vi "Test SMO Facade.vi"() -> ()   [LabVIEW 2019]
doc: "JKI State Machine Objects (SMO) 1.3.0.56\nJKI - JKI\nCopyright (c) 2017, JKI"
uses:
  SMO/SMO.lvclass
  SMO/Typedefs/SMOState --Enum.ctl
  Facade/SMOFacade.lvclass
panel:
  in  "Test Mismatch Inputs":bool
  out "Default Input":variant
  out "Method Prototype":string
  in  "Component URL":u16(ring) items=["System", "System/Subsystem"]
  in  "Invoke Method":bool
  in  "Public Methods":u16(ring) items=["CheckAccessibility", "Get GUID", "Get Name", "Get Qualified Name", "GetGUID", "GetName", "GetQualifiedName", "GetReserveState", "GetState", "Set Process Kill timeout", "WaitForStateChange", "is StateMachineObject", "isStateMachineObject"]
  out "Final Error":errorcluster
  out "return":variant
  out "Invoke Method Error":errorcluster
  # "Returns\n>>>>"
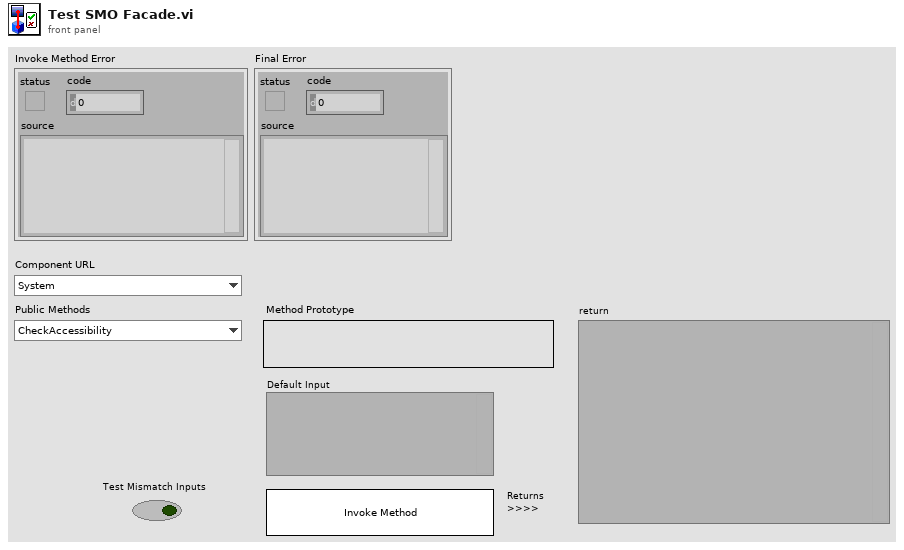
[diagram p1: front panel]
types:
  T1 = typedef "SMO.lvclass/Public Events.ctl" = cluster{"Error":refnum<user-event>, "State":refnum<user-event>, "Reserve State":refnum<user-event>}
  T2 = typedef "SMO.lvclass/SMOState --Enum.ctl" = enum16{"unknown", "Created", "Started", "Stopped"}
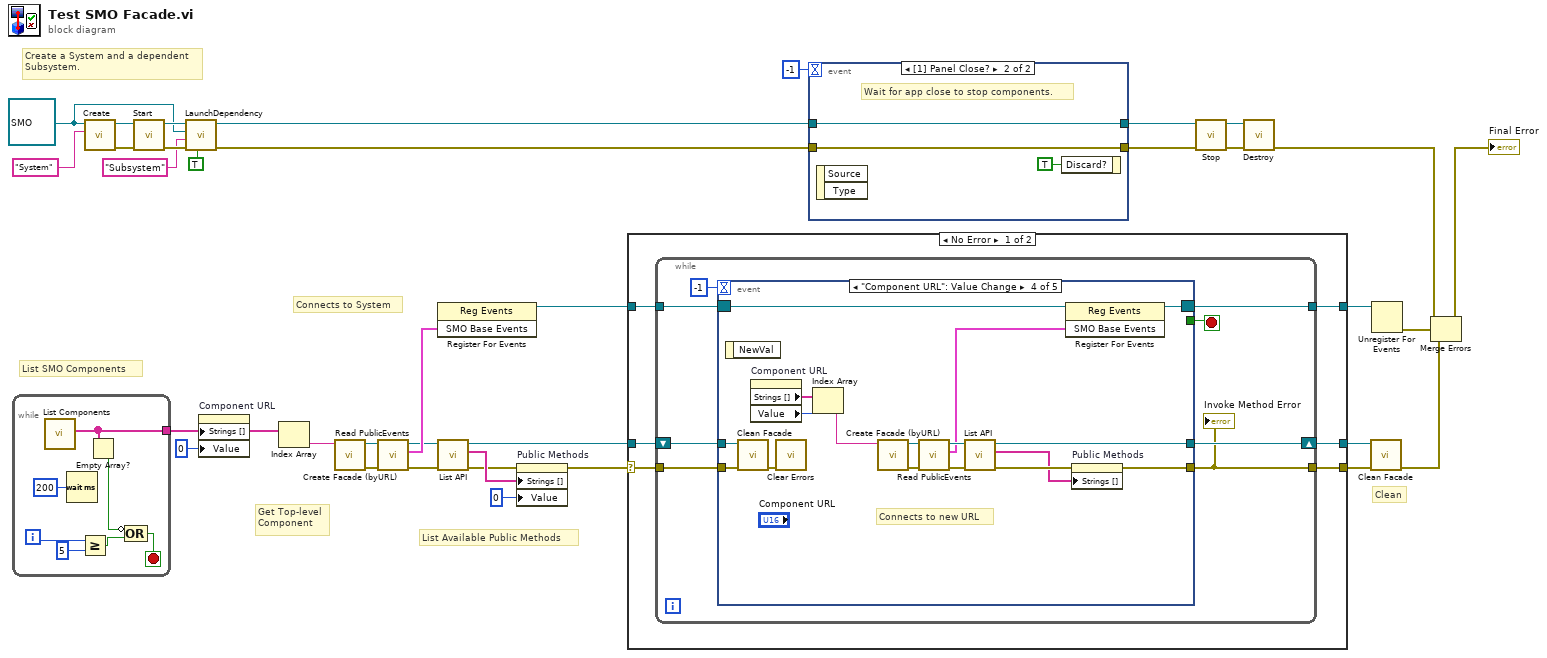
[diagram p0: block diagram]
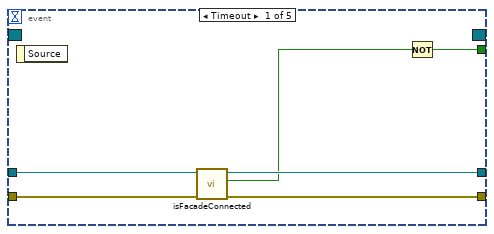
[diagram p2: hidden frame]
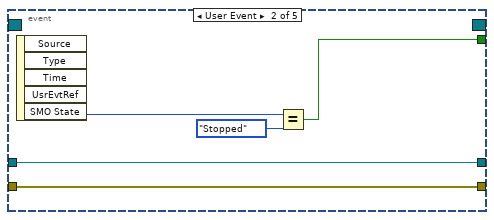
[diagram p3: hidden frame]
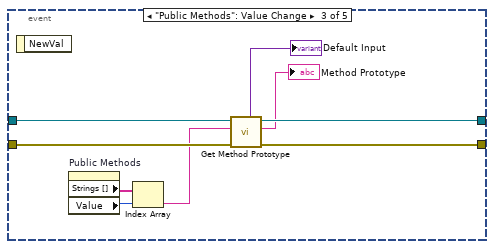
[diagram p4: hidden frame]
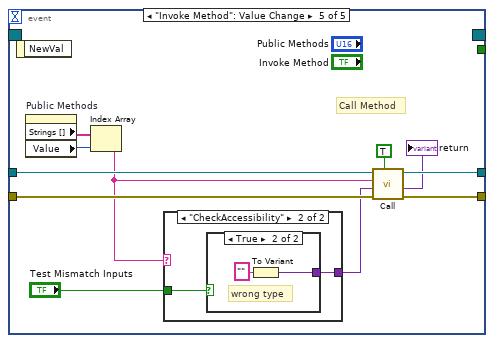
[diagram p5: hidden frame]
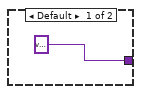
[diagram p6: hidden frame]
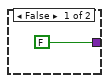
[diagram p7: hidden frame]
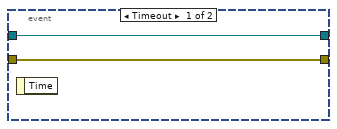
[diagram p9: hidden frame]
diagram:
  w15 = refnum<class "SMO.lvclass"> refnum ("SMO")
  # "List SMO Components"
  # "Get Top-level\nComponent"
  # "Connects to System"
  # "Clean"
  # "List Available Public Methods"
  # "Create a System and a dependent\nSubsystem."
  n1 = while {
    tunnel: [w37] -> w2
    i -> [w42]
    stop <- w39 stop-if-true
    n2 = call "List Components.vi"() -> ("Components"=w37:string[])  [unwired: 9 in, 2 out]
    n3 = Wait (ms)(milliseconds to wait=u32 200) -> ()  [unwired: 1 out]
    n4 = Greater Or Equal?(x=w42, y=5) -> (x >= y?=w40:bool)
    n5 = Empty Array?(array=w37) -> (empty?=w38:bool)
    n6 = Compound Arithmetic op=OR(invert w38, w40) -> (w39:bool)
  }
  n7 = call "Create.vi"("Subsystem Name (optional)"="System", "SMO"=w15) -> ("error out"=w23:errorcluster, "SMO out"=w24:refnum<class "SMO.lvclass">)  [unwired: 7 in, 1 out]
  n8 = call "Start.vi"("error in (no error)"=w23, "SMO"=w24) -> ("error out"=w21:errorcluster, "SMO out"=w22:refnum<class "SMO.lvclass">)  [unwired: 8 in]
  n9 = call "LaunchDependency.vi"("Shared Resource"=TRUE, "error in (no error)"=w21, "Dependency Name"="Subsystem" ("Subsystem Name (optional)"), "Dependency Type"=w15, "SMO in"=w22) -> ("error out"=w11:errorcluster, "SMO out"=w12:refnum<class "SMO.lvclass">)  [unwired: 3 in, 2 out]
  n10 = property on="Component URL" class="Ring (strict)"("Strings []"=w2, "Value"=u16 0) -> ()  [unwired: 2 in, 2 out]
  n11 = Index Array(array=w2) -> (element=w3:string)  [unwired: 1 in]
  n12 = call "Create Facade (byURL).vi"("URL"=w3) -> ("error out"=w4:errorcluster, "SMOFacade out"=w5:refnum<class "SMOFacade.lvclass">)  [unwired: 9 in]
  n13 = call "Read PublicEvents.vi"("error in (no error)"=w4, "SMOFacade in"=w5) -> ("error out"=w19:errorcluster, "SMO Base Events"=w18:T1, "SMOFacade out"=w17:refnum<class "SMOFacade.lvclass">)  [unwired: 7 in]
  n14 = register-events(w18) -> (reference out=w27:refnum<event-registration>)  [unwired: 2 in, 1 out]
  n15 = call "List API.vi"("error in (no error)"=w19, "SMOFacade in"=w17) -> ("error out"=w34:errorcluster, "Public API"=w35:string[], "SMOFacade out"=w36:refnum<class "SMOFacade.lvclass">)  [unwired: 7 in]
  n16 = property on="Public Methods" class="Ring (strict)"(error in=w34, "Strings []"=w35, "Value"=u16 0 ("Public Methods")) -> (error out=w6:errorcluster)  [unwired: 1 in, 1 out]
  n17 = case shown="No Error" w6 {
    selector: w6 -> [w44 w112]
    tunnel: w36 -> [w49 w113]
    tunnel: [w48 w113] -> w32
    tunnel: [w47 w112] -> w30
    tunnel: w27 -> [w46 w114]
    tunnel: [w45 w114] -> w26
    frame No Error {
      n18 = while {
        shift-right: [w54] -> w48
        shift-left: w49 -> [w55]
        tunnel: w44 -> [w53]
        tunnel: [w52] -> w47
        tunnel: w46 -> [w51]
        tunnel: [w50] -> w45
        stop <- w56 stop-if-true
        n19 = event shown="[3] \"Component URL\": Value Change" {
          selector: w51 -> [_ _ _ w83 _]
          dyn-events: [_ _ _ w82 _] -> w50
          timeout: -1 -> [_ _ _ _ _]
          tunnel: [w58 w64 _ _ _] -> w56
          tunnel: w55 -> [w61 w68 w72 w93 w105]
          tunnel: [w60 w68 w73 w89 w104] -> w54
          tunnel: [w62 w67 w74 w88 w102] -> w52
          tunnel: w53 -> [w63 w67 w75 w94 w103]
          event Timeout {
            n20 = event-data() -> ()  [unwired: 1 in, 1 out]
            n21 = call "isFacadeConnected.vi"("error in (no error)"=w63, "SMOFacade in"=w61) -> ("error out"=w62:errorcluster, "isConnected"=w59:bool, "SMOFacade out"=w60:refnum<class "SMOFacade.lvclass">)  [unwired: 7 in]
            n22 = Not(x=w59) -> (.not. x?=w58:bool)
          }
          event User Event {
            n23 = event-data() -> ("SMO State"=w66:T2)  [unwired: 1 in, 4 out]
            n24 = Equal?(x=w66, y=SMOState_--Enum."Stopped") -> (x = y?=w64:bool)
          }
          event "Public Methods": Value Change {
            n25 = event-data() -> ()  [unwired: 1 in, 1 out]
            n26 = property on="Public Methods" class="Ring (strict)"() -> ("Strings []"=w77:string[], "Value"=w76:u16)  [unwired: 2 in, 2 out]
            n27 = Index Array(array=w77, index=w76) -> (element=w71:string)
            n28 = call "Get Method Prototype.vi"("error in (no error)"=w75, "Method Name"=w71, "SMOFacade in"=w72) -> ("error out"=w74:errorcluster, "Method Prototype"=→"Method Prototype":string, "SMOFacade out"=w73:refnum<class "SMOFacade.lvclass">, "Default Input"=→"Default Input":variant)  [unwired: 4 in, 1 out]
          }
          event "Component URL": Value Change {
            # "Connects to new URL"
            n29 = event-data() -> ()  [unwired: 1 in, 1 out]
            n30 = call "Clean Facade.vi"("error in (no error)"=w94, "SMOFacade in"=w93) -> ("error out"=w92:errorcluster)  [unwired: 9 in]
            n31 = property on="Component URL" class="Ring (strict)"() -> ("Strings []"=w80:string[], "Value"=w79:u16)  [unwired: 2 in, 2 out]
            n32 = call <vilib>:"Clear Errors.vi"("error in (no error)"=w92) -> ()  [unwired: 5 in, 2 out]
            n33 = Index Array(array=w80, index=w79) -> (element=w78:string)
            n34 = call "Create Facade (byURL).vi"("URL"=w78) -> ("error out"=w86:errorcluster, "SMOFacade out"=w87:refnum<class "SMOFacade.lvclass">)  [unwired: 9 in]
            n35 = call "Read PublicEvents.vi"("error in (no error)"=w86, "SMOFacade in"=w87) -> ("error out"=w85:errorcluster, "SMO Base Events"=w81:T1, "SMOFacade out"=w84:refnum<class "SMOFacade.lvclass">)  [unwired: 7 in]
            n36 = call "List API.vi"("error in (no error)"=w85, "SMOFacade in"=w84) -> ("error out"=w91:errorcluster, "Public API"=w90:string[], "SMOFacade out"=w89:refnum<class "SMOFacade.lvclass">)  [unwired: 7 in]
            n37 = register-events(reference=w83, w81) -> (reference out=w82:refnum<event-registration>)  [unwired: 1 in, 1 out]
            n38 = property on="Public Methods" class="Ring (strict)"(error in=w91, "Strings []"=w90) -> (error out=w88:errorcluster)  [unwired: 1 in, 1 out]
          }
          event "Invoke Method": Value Change {
            # "Call Method"
            n39 = event-data() -> ()  [unwired: 1 in, 1 out]
            n40 = property on="Public Methods" class="Ring (strict)"() -> ("Strings []"=w99:string[], "Value"=w100:u16)  [unwired: 2 in, 2 out]
            n41 = Index Array(array=w99, index=w100) -> (element=w97:string)
            n42 = case shown="\"CheckAccessibility\"" w97 {
              tunnel: [variant ("variant") w108] -> w96
              tunnel: "Test Mismatch Inputs" -> [_ w107]
              frame Default {
              }
              frame "CheckAccessibility" {
                n43 = case shown="True" w107 {
                  tunnel: [FALSE w110] -> w108
                  frame False {
                  }
                  frame True {
                    # "wrong type"
                    n44 = To Variant(anything="") -> (Variant=w110:variant)
                  }
                }
              }
            }
            n45 = call "Call.vi"("Cache Ref (F)"=TRUE, "error in (no error)"=w103, "Inputs"=w96, "Method Name"=w97, "SMOFacade in"=w105) -> ("error out"=w102:errorcluster, "Outputs"=→"return":variant, "SMOFacade out"=w104:refnum<class "SMOFacade.lvclass">)  [unwired: 3 in, 1 out]
          }
        }
        "Invoke Method Error" <- w52
      }
    }
    frame Error {
    }
  }
  n46 = event shown="[1] Panel Close?" {
    selector: _ -> [_ _]
    dyn-events: _ -> [_ _]
    timeout: -1 -> [_ _]
    tunnel: w12 -> [w115 w118]
    tunnel: w11 -> [w116 w119]
    tunnel: [w116 w119] -> w9
    tunnel: [w115 w118] -> w10
    event Timeout {
      n47 = event-data() -> ()  [unwired: 1 in, 1 out]
    }
    event Panel Close? {
      # "Wait for app close to stop components."
      n48 = event-data() -> ()  [unwired: 1 in, 2 out]
      n49 = event-data("Discard?"=TRUE) -> ()  [unwired: 1 in, 1 out]
    }
  }
  n50 = call "Stop.vi"("error in (no error)"=w9, "SMO"=w10) -> ("error out"=w29:errorcluster, "SMO out"=w28:refnum<class "SMO.lvclass">)  [unwired: 8 in]
  n51 = call "Destroy.vi"("error in (no error)"=w29, "SMO"=w28) -> ("error out"=w8:errorcluster)  [unwired: 9 in]
  n52 = call "Clean Facade.vi"("error in (no error)"=w30, "SMOFacade in"=w32) -> ("error out"=w31:errorcluster)  [unwired: 9 in]
  n53 = Unregister For Events(event registration refnum=w26) -> (error out=w25:errorcluster)  [unwired: 1 in]
  n54 = Merge Errors(w8, w25, w31) -> (→"Final Error":errorcluster)
